vi "已贴标签B.vi"(3 "2D_Code":string) -> ()   [LabVIEW 2014]
panel:
  out "结果字符串":string
  out "error out":errorcluster
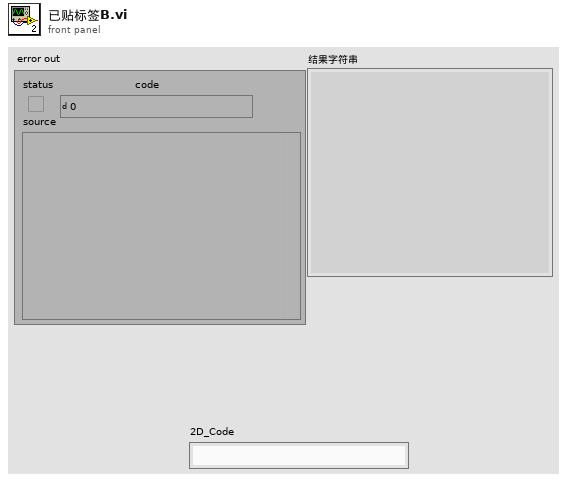
[diagram p1: front panel]
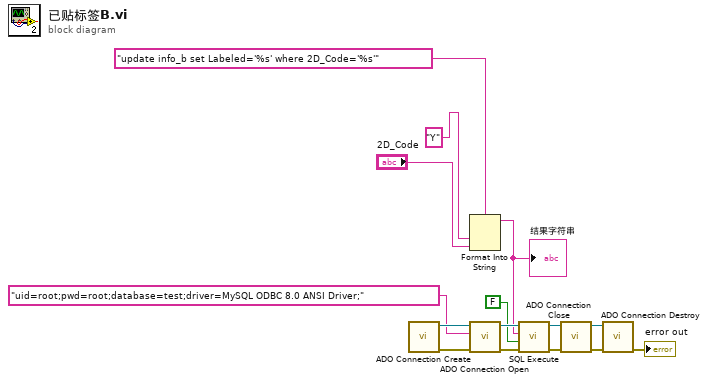
[diagram p0: block diagram]
diagram:
  n1 = call "ADO Connection Create.vi"() -> ("error out"=w14:errorcluster, "ADODB._Connection Out"=w15:refnum<k7>)  [unwired: 10 in]
  n2 = Format Into String(format string="update info_b set Labeled='%s' where 2D_Code='%s'" ("Command Text"), "Y" ("输入 1"), "2D_Code") -> (resulting string=w3:string)  [unwired: 2 in, 1 out]
  "结果字符串" <- w3
  n3 = call "ADO Connection Open.vi"("error in (no error)"=w14, "ConnectionString"="uid=root;pwd=root;database=test;driver=MySQL ODBC 8.0 ANSI Driver;", "ADODB._Connection In"=w15) -> ("error out"=w12:errorcluster, "ADODB._Connection Out"=w13:refnum<k7>)  [unwired: 7 in]
  n4 = call "SQL Execute.vi"("error in (no error)"=w12, "Return Data (T)"=FALSE, "Command Text"=w3, "ADODB._Connection In"=w13) -> ("error out"=w10:errorcluster, "ADODB._Connection Out"=w11:refnum<k7>)  [unwired: 4 in, 2 out]
  n5 = call "ADO Connection Close.vi"("error in (no error)"=w10, "ADODB._Connection In"=w11) -> ("error out"=w8:errorcluster, "ADODB._Connection Out"=w9:refnum<k7>)  [unwired: 8 in]
  n6 = call "ADO Connection Destroy.vi"("error in (no error)"=w8, "ADODB._Connection In"=w9) -> ("error out"=→"error out":errorcluster)  [unwired: 9 in]
